vi "Error Merging.vi"(1 "error 2 in":errorcluster, 2 "errors in":errorcluster[](array[cluster]), 3 "error 1 in":errorcluster) -> (0 "error out":errorcluster)   [LabVIEW 2013]
doc: "This vi will return the first error encountered in the list of error clusters. If \"error 1 in\" contains an error, this will be returned in \"error out\". If \"error 1 in\" does not contain an error, the first error in the \"errors in\" array will be returned. If none of these error clusters contains and error, then \"error 2 in\" will be returned in \"error out\".\n\nCopyright © 1998 by Mark Naley. All rights reserved."
panel:
  # "Copyright © 1998 by Mark Naley.  All rights reserved.\nAuthor makes no warranties or guarantees related to performance of the software.\nUSE AT YOUR OWN RISK."
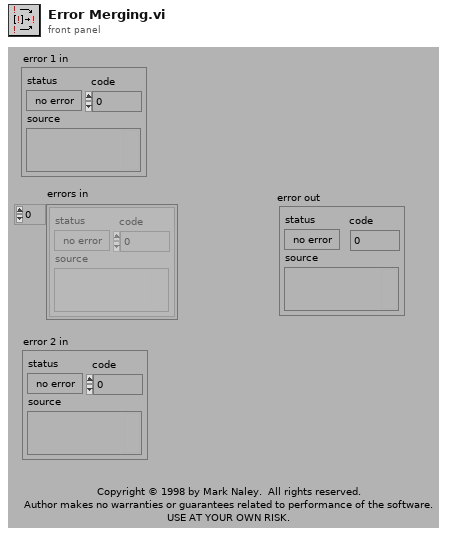
[diagram p1: front panel]
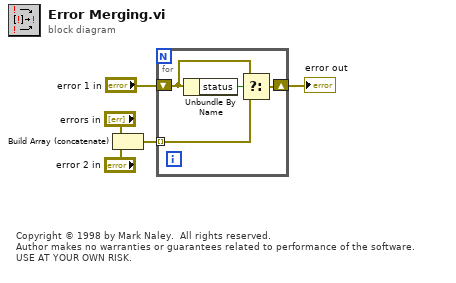
[diagram p0: block diagram]
diagram:
  # "Copyright © 1998 by Mark Naley.  All rights reserved.\nAuthor makes no warranties or guarantees related to performance of the software.\nUSE AT YOUR OWN RISK."
  n1 = Build Array (concatenate)("errors in", "error 2 in") -> (w1:errorcluster[])
  n2 = for {
    shift-right: [w7] -> w4
    shift-left: "error 1 in" -> [w9]
    tunnel: w1 -> [w6] mode=indexing
    n3 = Unbundle By Name(w9) -> ("status"=w8:bool)
    n4 = Select(t=w9, s=w8, f=w6) -> (s? t:f=w7:errorcluster)
  }
  "error out" <- w4
